vi "Write Binary File.vi"() -> ()   [LabVIEW 2023]
doc: "Writes an array of data into a byte stream binary file. By default, the VI is configured to write 8-byte (data type DBL) Little Endian Data. To modify the way sample data is written to the file, change the Byte Order and convert the array of data (default DBL) into an I8(1-byte), I16(2-byte), or I32(4-byte) using the VIs found in the Programming >> Numeric >> Conversion Palette. Use the Read Binary File VI to read the file."
panel:
  out "Data Written to File":dbl[](graph)
  # "Overview: Demonstrates the use of the File I/O functions to write data to a binary file.\nInstructions:\n1. Run this VI.\n2. Open Read Binary File.vi and follow the instructions on its front panel."
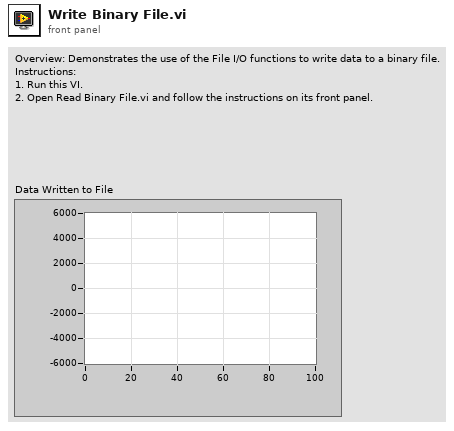
[diagram p1: front panel]
types:
  T1 = enum16{"open", "replace", "create", "open or create", "replace or create", "replace or create with confirmation"}
  T2 = enum16{"big-endian, network order", "native, host order", "little-endian"}
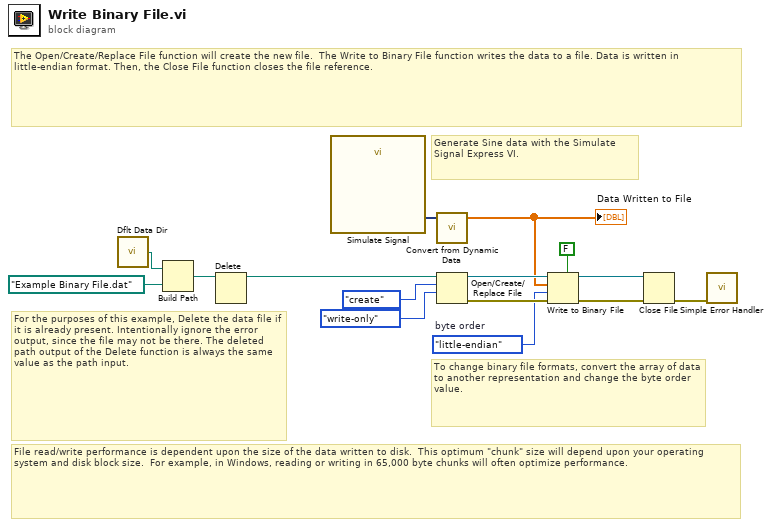
[diagram p0: block diagram]
diagram:
  w8 = T2."little-endian"  # byte order
  # "File read/write performance is dependent upon the size of the data written to disk.  This optimum \"chunk\" size will depend upon your operating system and disk block size.  For example, in Windows, reading or writing in 65,000 byte chunks will often optimize performance."
  # "To change binary file formats, convert the array of data to another representation and change the byte order value."
  # "For the purposes of this example, Delete the data file if it is already present. Intentionally ignore the error output, since the file may not be there. The deleted path output of the Delete function is always the same value as the path input."
  # "Generate Sine data with the Simulate Signal Express VI."
  # "The Open/Create/Replace File function will create the new file.  The Write to Binary File function writes the data to a file. Data is written in little-endian format. Then, the Close File function closes the file reference."
  n1 = call <vilib>:"Dflt Data Dir.vi"() -> ("App:Default Data Directory"=w4:path)
  n2 = Build Path(base path=w4, name or relative path=path "Example Binary File.dat" ("default name")) -> (appended path=w2:path)
  n3 = Delete(path (use dialog)=w2) -> (deleted path=w1:path)  [unwired: 4 in, 2 out]
  n4 = call "Simulate Signal"() -> ("Sine"=w6:dynamicdata)  [unwired: 14 in, 1 out]
  n5 = call "Convert from Dynamic Data"("Dynamic Data Type"=w6) -> ("Array"=w5:dbl[])  [unwired: 3 in]
  "Data Written to File" <- w5
  n6 = Open/Create/Replace File(file path (use dialog)=w1, operation (0:open)=T1."create", access (0:read/write)=enum16{"read/write", "read-only", "write-only"}."write-only") -> (refnum out=w11:refnum<file>, error out=w12:errorcluster)  [unwired: 3 in, 1 out]
  n7 = Write to Binary File(file (use dialog)=w11, data=w5, error in=w12, 5:FALSE ("prepend array or string size? (T)"), 9:w8) -> (refnum out=w15:refnum<file>, error out=w14:errorcluster)  [unwired: 1 in, 1 out]
  n8 = Close File(refnum=w15, error in=w14) -> (error out=w13:errorcluster)  [unwired: 1 out]
  n9 = call <vilib>:"Simple Error Handler.vi"("error in (no error)"=w13) -> ()  [unwired: 4 in, 5 out]
